vi "fahrenheit_to_celsius.vi"(1 "Fahrenheit":sgl format="%#.1f") -> (0 "Celsius":sgl format="%#.1f")   [LabVIEW 2012]
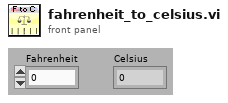
[diagram p1: front panel]
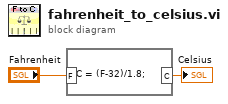
[diagram p0: block diagram]
diagram:
  n1 = formula code="C = (F-32)/1.8;"("F"="Fahrenheit") -> ("C"=→"Celsius":dbl)
